vi "InitializeFpgaBurstMode.vi"(8 "error in (no error)":errorcluster, 11 "923x Acquisition Config":T1={"Acq"=FALSE, "NumberOfModules"=0, "Dynamic FPGA VI Ref"=refnum, "KeyphasorX3"=[], "FixedSizeX32"={"EnabledChannels"=[], "Sensitivity"=[], "InputConfig"=[]}, "SamplingInfo"={"Number of Channels"=4, "Sampling Rate"=4.0, "Channels"=[], "Units"=[], "Offsets"=[]}, "Normal Mode Sample Rate"=0.0, "BlockSize (sec)"=0.0, "Samples To Read (per chan)"=0, "RunningAcquisitionLength"=0.0, "Settling Time"=0.0, "Waveform Groups"=[], "Acquisition Block Number"=0, "Device Name"="", "ValidConfig"=FALSE, "Last Dynamic Module"="", "HighPassFilterState"=[], "Low Frequency Cutoff"=[], "BurstMode"={"Acquisition Time"=0.0, "Sample Rate"=0.0}} {"HighPassFilterState"."Filter State" format="%.2f"; "HighPassFilterState"."IIR Filter Cluster"."Forward Coefficients" format="%.2f"; "HighPassFilterState"."IIR Filter Cluster"."Reverse Coefficients" format="%.2f"; "FixedSizeX32"."InputConfig" items=["AC Coupled", "DC Coupled", "IEPE AC Coupled"]}) -> (0 "error out":errorcluster, 1 "start acquisition?":bool, 2 "dynamic FPGA VI reference":refnum<k20>, 3 "923x Acquisition Config out":T1={"Acq"=FALSE, "NumberOfModules"=0, "Dynamic FPGA VI Ref"=refnum, "KeyphasorX3"=[], "FixedSizeX32"={"EnabledChannels"=[], "Sensitivity"=[], "InputConfig"=[]}, "SamplingInfo"={"Number of Channels"=4, "Sampling Rate"=4.0, "Channels"=[], "Units"=[], "Offsets"=[]}, "Normal Mode Sample Rate"=0.0, "BlockSize (sec)"=0.0, "Samples To Read (per chan)"=0, "RunningAcquisitionLength"=0.0, "Settling Time"=0.0, "Waveform Groups"=[], "Acquisition Block Number"=0, "Device Name"="", "ValidConfig"=FALSE, "Last Dynamic Module"="", "HighPassFilterState"=[], "Low Frequency Cutoff"=[], "BurstMode"={"Acquisition Time"=0.0, "Sample Rate"=0.0}} {"HighPassFilterState"."Filter State" format="%.2f"; "HighPassFilterState"."IIR Filter Cluster"."Forward Coefficients" format="%.2f"; "HighPassFilterState"."IIR Filter Cluster"."Reverse Coefficients" format="%.2f"; "FixedSizeX32"."InputConfig" items=["AC Coupled", "DC Coupled", "IEPE AC Coupled"]})   [LabVIEW 2017, in "CmsAcquisition.lvlib"]
doc: "Initializes the acquisition of the dynamic channels with the RIO Wfm API."
uses:
  <vilib>/addons/InsightCM/Devices/Shared/Cms/CmsAcquisition/CmsAcquisition.lvlib
  <vilib>/addons/InsightCM/Devices/Shared/Cms/CmsAcquisition/controls/Configuration.ctl
  <vilib>/addons/InsightCM/Devices/Shared/Cms/CmsAcquisition/controls/TachometerConfig.ctl
  <vilib>/addons/InsightCM/Devices/Shared/Cms/CmsAcquisition/controls/FixedSizeArrays.ctl
  <vilib>/LabVIEW Targets/FPGA/cRIO/shared/nicrio_ModuleControls/nicrio_cRIO-9232_ConfigModeRing.ctl
  <vilib>/addons/InsightCM/Devices/Shared/Cms/cRIOWfmAcq/subVIs/RIO Wfm Cust Ctrls/rwfm_SamplingInfo.ctl
  <vilib>/addons/InsightCM/Devices/Shared/Cms/CmsAcquisition/controls/Group.ctl
  <vilib>/addons/InsightCM/Devices/Shared/Cms/CmsAcquisition/controls/Channel.ctl
  <vilib>/addons/InsightCM/Utilities/Analysis/Vibration/controls/HighPassFilterState.ctl
  <vilib>/addons/InsightCM/Devices/Shared/Cms/CmsAcquisition/controls/BurstMode.ctl
  <vilib>/Utility/error.llb/Error Cluster From Error Code.vi
  <vilib>/rvi/errors/niLvFpgaAdjustHostInterfaceError.vi
  <vilib>/rvi/interface/nirviReadWriteControl/nirviReadWriteControl.xnode
  <vilib>/addons/InsightCM/Devices/Shared/Cms/cRIOWfmAcq/cRIOWfmLib.lvlib
  NiFpgaLv.dll
  <vilib>/rvi/interface/Simulation/niFpgaSimulationCallBeginRW.vi
  <vilib>/addons/InsightCM/Utilities/Analysis/Vibration/VibrationAnalysisFunctions.lvlib
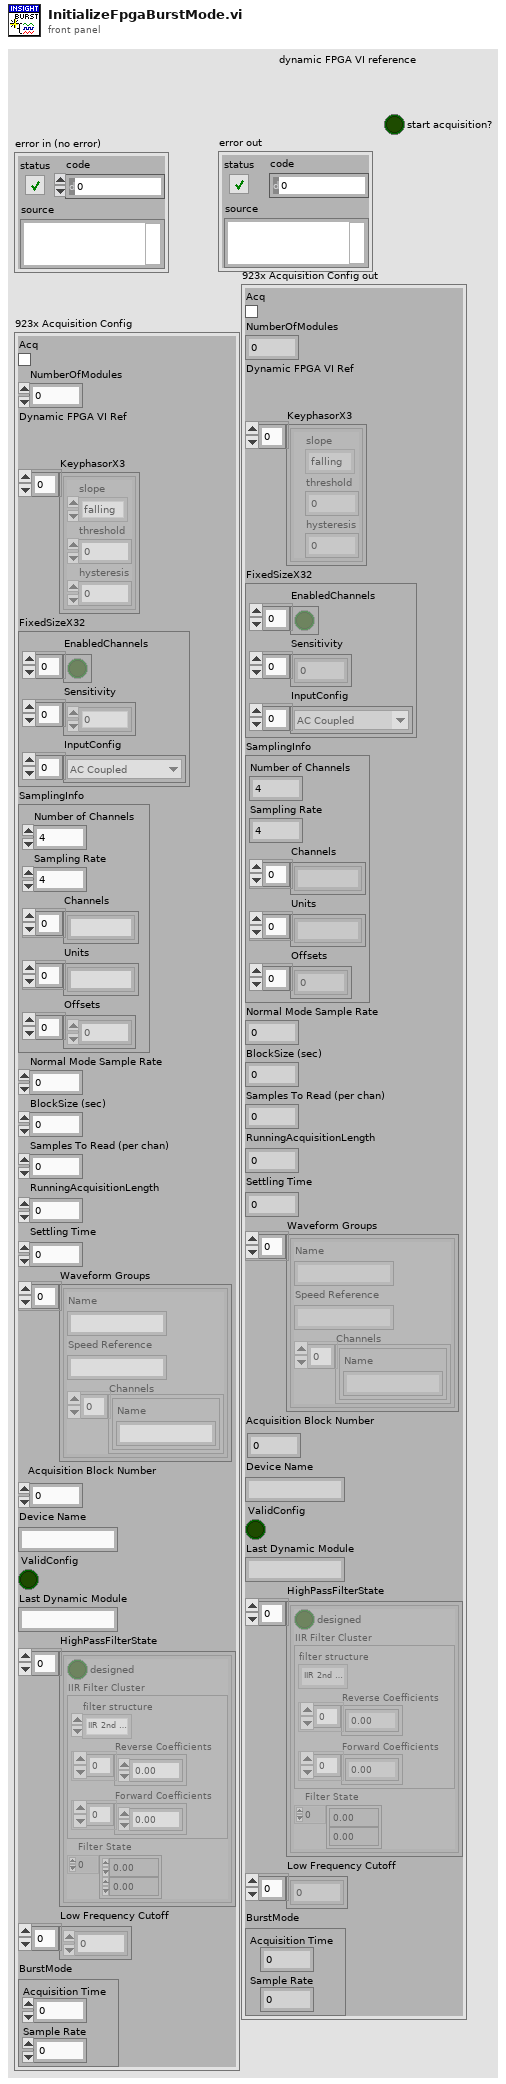
[diagram p1: front panel]
types:
  T1 = typedef "CmsAcquisition.lvlib/Configuration.ctl" = cluster{"Acq":bool, "NumberOfModules":i16, "Dynamic FPGA VI Ref":refnum<k20>, "KeyphasorX3":T2[], "FixedSizeX32":T3, "SamplingInfo":T5, "Normal Mode Sample Rate":dbl, "BlockSize (sec)":dbl, "Samples To Read (per chan)":i32, "RunningAcquisitionLength":dbl, "Settling Time":dbl, "Waveform Groups":T6[], "Acquisition Block Number":i32, "Device Name":string, "ValidConfig":bool, "Last Dynamic Module":string, "HighPassFilterState":T8[], "Low Frequency Cutoff":dbl[], "BurstMode":T9}
  T2 = typedef "CmsAcquisition.lvlib/TachometerConfig.ctl" = cluster{"slope":enum16{"falling", "rising"}, "threshold":dbl, "hysteresis":dbl}
  T3 = typedef "CmsAcquisition.lvlib/FixedSizeArrays.ctl" = cluster{"EnabledChannels":bool[], "Sensitivity":dbl[], "InputConfig":T4[]}
  T4 = typedef "nicrio_cRIO-9232_ConfigModeRing.ctl" = u8
  T5 = typedef "cRIOWfmLib.lvlib/rwfm_SamplingInfo.ctl" = cluster{"Number of Channels":i32, "Sampling Rate":dbl, "Channels":string[], "Units":string[], "Offsets":sgl[]}
  T6 = typedef "CmsAcquisition.lvlib/Group.ctl" = cluster{"Name":string, "Speed Reference":string, "Channels":T7[]}
  T7 = typedef "CmsAcquisition.lvlib/Channel.ctl" = cluster{"Name":string}
  T8 = typedef "VibrationAnalysisFunctions.lvlib/HighPassFilterState.ctl" = cluster{"designed":bool, "IIR Filter Cluster":cluster{"filter structure":enum32{"IIR 2nd Order", "IIR 4th Order"}, "Reverse Coefficients":dbl[], "Forward Coefficients":dbl[]}, "Filter State":dbl[]}
  T9 = typedef "CmsAcquisition.lvlib/BurstMode.ctl" = cluster{"Acquisition Time":dbl, "Sample Rate":dbl}
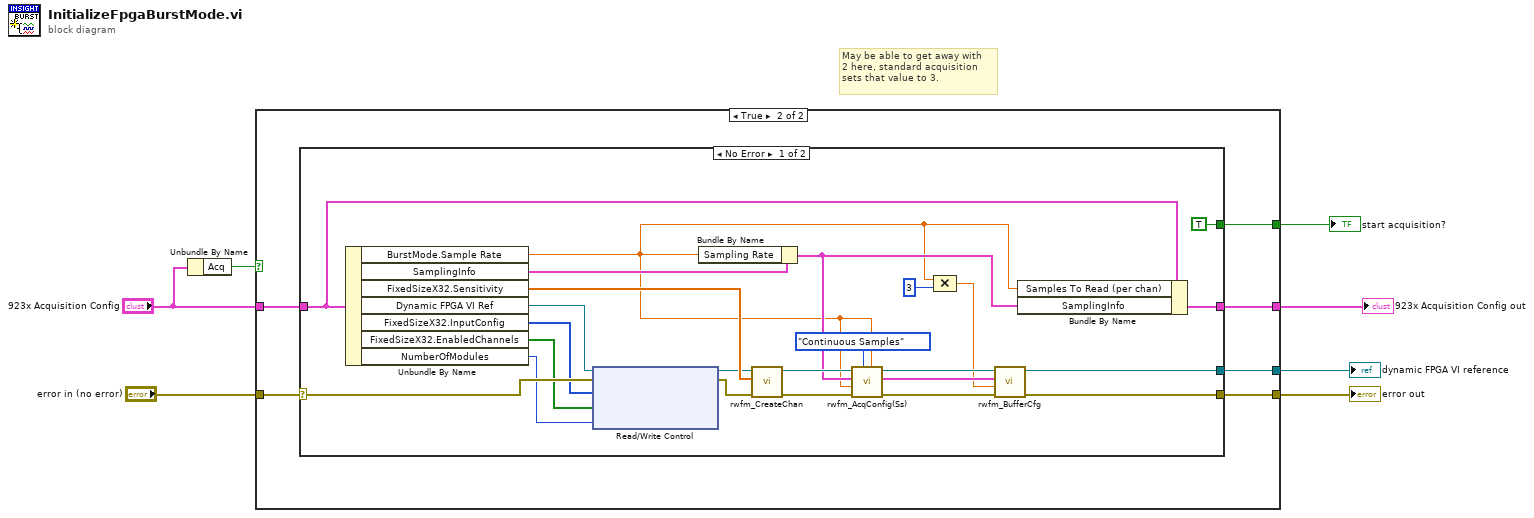
[diagram p0: block diagram]
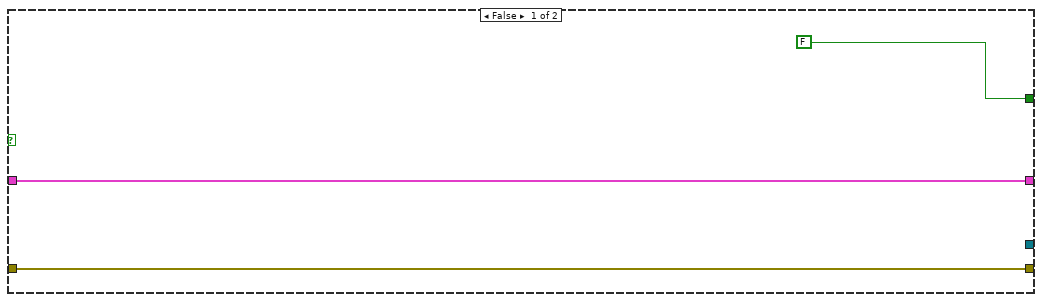
[diagram p2: hidden frame]
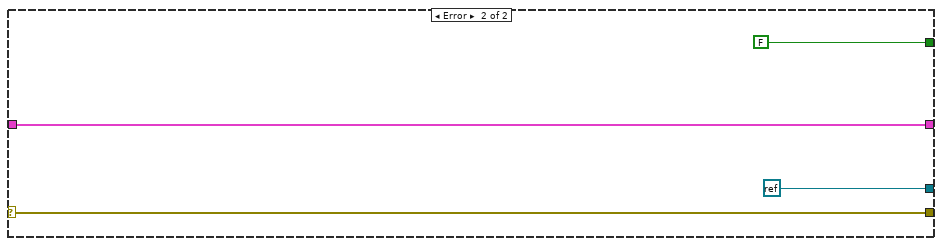
[diagram p3: hidden frame]
diagram:
  # "May be able to get away with\n2 here, standard acquisition\nsets that value to 3."
  n1 = Unbundle By Name("923x Acquisition Config") -> ("Acq"=w2:bool)
  n2 = case shown="True" w2 {
    tunnel: "923x Acquisition Config" -> [w8 w16]
    tunnel: [w10 w15] -> w7
    tunnel: "error in (no error)" -> [w10 w14]
    tunnel: [_ w13] -> w5
    tunnel: [FALSE w12] -> w4
    tunnel: [w8 w11] -> w1
    frame False {
    }
    frame True {
      n3 = case shown="No Error" w14 {
        selector: w14 -> [w39 w43]
        tunnel: w16 -> [w20 w41]
        tunnel: [w26 w43] -> w15
        tunnel: [w24 refnum<k0> refnum] -> w13
        tunnel: [TRUE FALSE] -> w12
        tunnel: [w19 w41] -> w11
        frame No Error {
          n4 = Unbundle By Name(w20) -> ("BurstMode.Sample Rate"=w17:dbl, "SamplingInfo"=w28:T5, "FixedSizeX32.Sensitivity"=w40:dbl[], "Dynamic FPGA VI Ref"=w38:refnum<k20>, "FixedSizeX32.InputConfig"=w30:T4[], "FixedSizeX32.EnabledChannels"=w31:bool[], "NumberOfModules"=w32:i16)
          n5 = xnode "Read/Write Control"("FPGA VI Reference In"=w38, "error in"=w39, "Input Config Array"=w30, "Enable Chan Array"=w31, "Number of Modules"=w32) -> ("FPGA VI Reference Out"=w37:refnum<k20>, "error out"=w35:errorcluster)
          n6 = Bundle By Name(cluster=w28, "Sampling Rate"=w17) -> (w18:T5)
          n7 = call <vilib>:"rwfm_CreateChan.vi"("error in"=w35, "Sensitivity"=w40, "Dynamic FPGA VI Reference"=w37) -> ("error out"=w33:errorcluster, "Dynamic FPGA VI Reference"=w34:refnum<k20>)  [unwired: 7 in]
          n8 = call <vilib>:"rwfm_AcqConfig(Ss).vi"("Samples per Channel"=w17, "Sample Mode"=enum16{"Finite Samples", "Continuous Samples"}."Continuous Samples", "error in"=w33, "Sample Rate S/s"=w17, "Sampling Info In"=w18, "Dynamic FPGA Ref"=w34) -> ("error out"=w27:errorcluster, "Sampling Info Out"=w23:T5, "Dynamic FPGA Ref Out"=w25:refnum<k20>)  [unwired: 2 in, 1 out]
          n9 = Compound Arithmetic op=MULTIPLY(w17, 3 ("value")) -> (w21:dbl)
          n10 = call <vilib>:"rwfm_BufferCfg.vi"("error in"=w27, "Buffer Size [Samps per Chan]"=w21, "Sampling Info In"=w23, "Dynamic FPGA VI Reference"=w25) -> ("error out"=w26:errorcluster, "Dynamic FPGA VI Reference"=w24:refnum<k20>)  [unwired: 4 in, 2 out]
          n11 = Bundle By Name(cluster=w20, "Samples To Read (per chan)"=w17, "SamplingInfo"=w18) -> (w19:T1)
        }
        frame Error {
        }
      }
    }
  }
  "error out" <- w7
  "dynamic FPGA VI reference" <- w5
  "start acquisition?" <- w4
  "923x Acquisition Config out" <- w1
